vi "readIMU TEST.vi"() -> ()   [LabVIEW 2019]
uses:
  <vilib>/rvi/Emulation/niFpgaGetClockAttributes.vi
  <vilib>/rvi/Emulation/niFpgaSctlEmulationGetInTimedLoop.vi
  <vilib>/rvi/Emulation/niFpgaEmulationReportErrorSimple.vi
  <vilib>/rvi/Emulation/niFpgaCriticalErrorInLSC.vi
panel:
  out "az":fxp<+/-,32,16>
  in  "stop":bool
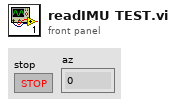
[diagram p1: front panel]
types:
  T1 = typedef "IMU Config.ctl" = cluster{"Accelerometer Bias":i16[], "Accelerometer Scale":i16, "Gyro Bias":i16[], "Gyro Scale":i16}
  T2 = typedef "SPI Config.ctl" = cluster{"MXP Port":enum16{"A", "B"}, "Device":enum16{"CAN", "ENC", "IMU1", "IMU2"}, "CPOL":bool}
  T3 = cluster{fxp<+/-,32,16>, fxp<+/-,32,16>, fxp<+/-,32,16>, fxp<+/-,32,16>, fxp<+/-,32,16>, fxp<+/-,32,16>}
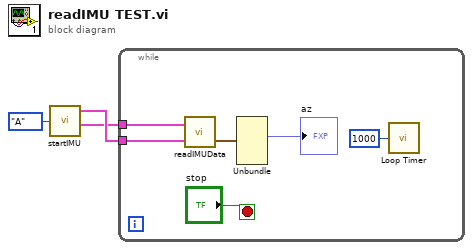
[diagram p0: block diagram]
diagram:
  n1 = call "startIMU.vi"("MXP Port"=enum16{"A", "B"}."A") -> ("IMU Config Out"=w3:T1, "IMU1 SPI Config"=w2:T2)  [unwired: 1 out]
  n2 = while {
    tunnel: w3 -> [w9]
    tunnel: w2 -> [w8]
    stop <- "stop" stop-if-true
    n3 = call "readIMUData.vi"("IMU Config In"=w9, "SPI Config In"=w8) -> ("Data Out"=w7:T3)  [unwired: 1 out]
    n4 = Unbundle(w7) -> (→"az":fxp<+/-,32,16>)  [unwired: 5 out]
    n5 = call "Loop Timer"("Count(mSec)"=u32 1000) -> ()  [unwired: 1 out]
  }
